vi "FIFO.vi"(10 "Fi":dbl, 11 "FIFO size":i32) -> (2 "Array out":dbl[](array[numeric]), 3 "Fo":dbl)   [LabVIEW 2013]
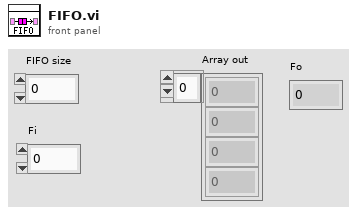
[diagram p1: front panel]
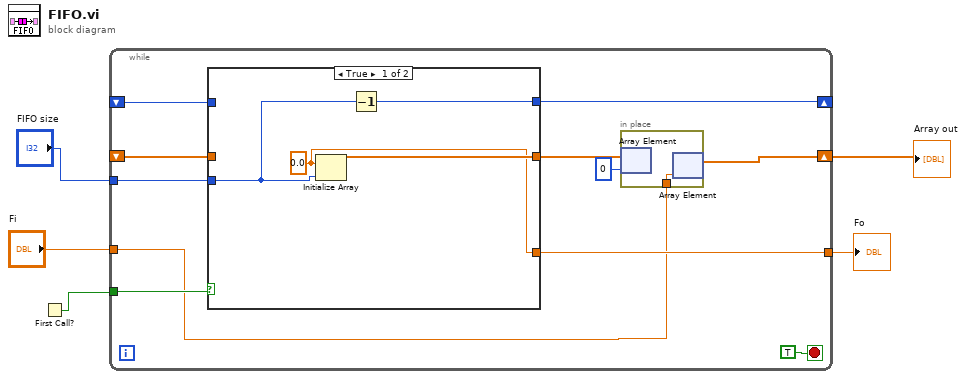
[diagram p0: block diagram]
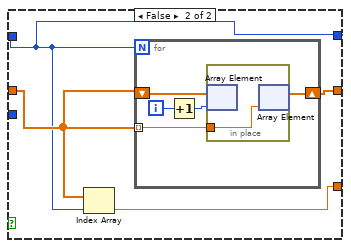
[diagram p2: hidden frame]
diagram:
  n1 = First Call?() -> (First Call?: T/F=w5:bool)
  n2 = while {
    tunnel: w5 -> [w14]
    shift-right: [w9] -> w1
    shift-left: _ -> [w16]
    shift-right: [w12] -> _
    shift-left: _ -> [w15]
    tunnel: "FIFO size" -> [w11]
    tunnel: "Fi" -> [w7]
    tunnel: [w8] -> w2
    stop <- TRUE stop-if-true
    n3 = case shown="True" w14 {
      tunnel: w16 -> [_ w24]
      tunnel: [w20 w25] -> w10
      tunnel: w15 -> [_ w23]
      tunnel: [w21 w23] -> w12
      tunnel: w11 -> [w19 _]
      tunnel: [w18 w22] -> w8
      frame True {
        w18 = 0.0 ("element")
        n4 = Initialize Array(w18, w19) -> (w20:dbl[])
        n5 = Decrement(x=w19) -> (x-1=w21:i32)
      }
      frame False {
        n6 = Index Array(array=w24, index=w23) -> (element=w22:dbl)
        n7 = for {
          N: w23 -> [_]
          shift-right: [w27] -> w25
          shift-left: w24 -> [w26]
          tunnel: w24 -> [w28] mode=indexing
          i -> [w30]
          n8 = Increment(x=w30) -> (x+1=w29:i32)
          n9 = in-place {
            in-place-border: w28 -> [w31]
            n10 = in-place-array #1(w26, w29) -> ()  [unwired: 1 out]
            n11 = in-place-array #1(w31) -> (w27:dbl[])  [unwired: 1 out]
          }
        }
      }
    }
    n12 = in-place {
      in-place-border: w7 -> [w17]
      n13 = in-place-array #2(w10, 0) -> ()  [unwired: 1 out]
      n14 = in-place-array #2(w17) -> (w9:dbl[])  [unwired: 1 out]
    }
  }
  "Array out" <- w1
  "Fo" <- w2
